vi "CL3IF_GetStorageIndex.vi"(8 "error in":errorcluster {"code" format="%x"}, 10 "selectedIndex":T1, 11 "deviceId":i32) -> (0 "error out":errorcluster {"code" format="%x"}, 2 "index":u32)   [LabVIEW 2020, in "Keyence CL-3000.lvlib"]
doc: "This function is used to get the data stored on the device."
uses:
  Keyence CL-3000.lvlib
  enums/CL3IF_SELECTED_INDEX.ctl
  Private/enums/Function Name.ctl
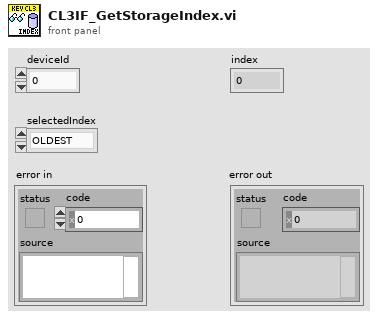
[diagram p1: front panel]
types:
  T1 = typedef "Keyence CL-3000.lvlib/CL3IF_SELECTED_INDEX.ctl" = enum16{"OLDEST", "NEWEST"}
  T2 = typedef "Keyence CL-3000.lvlib/Function Name.ctl" = enum16{"Initialize", "Close", "CL3IF_GetMeasurementData", "CL3IF_GetTrendIndex", "CL3IF_GetTrendData", "CL3IF_GetStorageIndex", "CL3IF_GetStorageData", "CL3IF_AutoZeroMulti", "CL3IF_AutoZeroGroup", "CL3IF_TimingMulti", "CL3IF_TimingGroup", "CL3IF_ResetMulti", "CL3IF_ResetGroup", "CL3IF_LightControl", "CL3IF_MeasurementControl", "CL3IF_SwitchProgram", "CL3IF_GetProgramNo", "CL3IF_StartStorage", "CL3IF_StopStorage", "CL3IF_ClearStorageData", "CL3IF_GetPulseCount", "CL3IF_ResetPulseCount", "CL3IF_GetLightWaveform"}
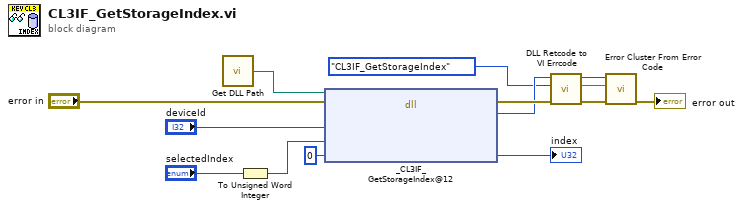
[diagram p0: block diagram]
diagram:
  n1 = call "Get DLL Path.vi"() -> ("DLL Path"=w10:path)  [unwired: 1 in]
  n2 = To Unsigned Word Integer(number="selectedIndex") -> (unsigned 16bit integer=w5:u16)
  n3 = dll-call lib="C:/Program Files (x86)/National Instruments/LabVIEW 2018/instr.lib/Keyence CL-3000/CL3_IF.dll" fn="_CL3IF_GetStorageIndex@12"(path in=w10, error in="error in", "deviceId"="deviceId", "selectedIndex"=w5, "index"=u32 0) -> (error out=w9:errorcluster, "RC"=w8:i32, "index"=→"index":u32)  [unwired: 3 in, 1 out]
  n4 = call "DLL Retcode to VI Errcode.vi"("error in (no error)"=w9, "Function Name"=Function_Name."CL3IF_GetStorageIndex", "DLL Retcode"=w8) -> ("error out"=w14:errorcluster, "ErrorMessage"=w2:string, "VI Errcode"=w13:i32)  [unwired: 6 in]
  n5 = call <vilib>:"Error Cluster From Error Code.vi"("error in (no error)"=w14, "error message (\"\")"=w2, "error code (0)"=w13) -> ("error out"=→"error out":errorcluster)  [unwired: 6 in]
